vi "Slave.vi"() -> ()   [LabVIEW 2014]
panel:
  in  "stop":bool
  in  "data in":bool
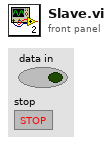
[diagram p1: front panel]
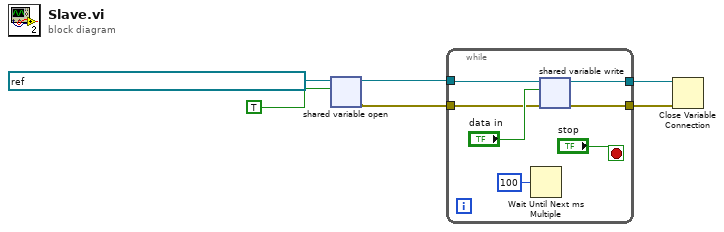
[diagram p0: block diagram]
diagram:
  n1 = shared-variable-open(refnum<k21> "ni.var.psp://ni-myrio-gsiep/DataBase_Slave/000001" ("shared variable refnum in"), TRUE ("data type")) -> (w4:refnum<k21>, w3:errorcluster)  [unwired: 2 in]
  n2 = while {
    tunnel: w4 -> [w13]
    tunnel: w3 -> [w11]
    tunnel: [w10] -> w2
    tunnel: [w9] -> w1
    stop <- "stop" stop-if-true
    n3 = Wait Until Next ms Multiple(millisecond multiple=u32 100) -> ()  [unwired: 1 out]
    n4 = shared-variable-write(w13, w11, "data in") -> (w10:refnum<k21>, w9:errorcluster)
  }
  n5 = Close Variable Connection(8:w1, 11:w2) -> ()  [unwired: 1 out]
